vi "Spray_set_amplitude.vi"(1 "input 1":string, 3 "error in (no error)":errorcluster) -> (10 "error out":errorcluster)   [LabVIEW 2015]
uses:
  <vilib>/httpClient/LabVIEWHTTPClient.lvlib
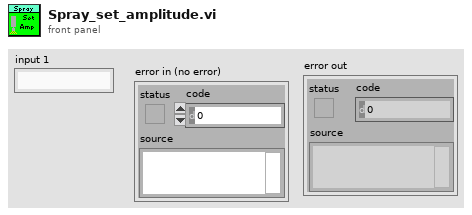
[diagram p1: front panel]
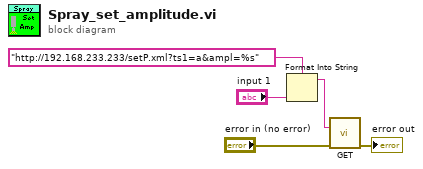
[diagram p0: block diagram]
diagram:
  n1 = Format Into String(format string="http://192.168.233.233/setP.xml?ts1=a&ampl=%s" ("url"), "input 1") -> (resulting string=w1:string)  [unwired: 2 in, 1 out]
  n2 = call <vilib>:"GET.vi"("url"=w1, "error in (no error)"="error in (no error)") -> ("error out"=→"error out":errorcluster)  [unwired: 10 in, 3 out]
